vi "asset.update_set_name.vi"(8 "error in":errorcluster, 11 "AssetUpdateStaging in":refnum<class "AssetUpdateStaging.lvclass">) -> (0 "error out":errorcluster, 3 "AssetUpdateStaging out":refnum<class "AssetUpdateStaging.lvclass">)   [LabVIEW 2020, in "AssetUpdateStaging.lvclass"]
doc: "Stages a new name for the asset being updated."
uses:
  AssetUpdateStaging.lvclass
  AssetUpdateStaging.lvclass/AssetUpdateStaging.ctl
  client.lvlib
panel:
  in  "name":string
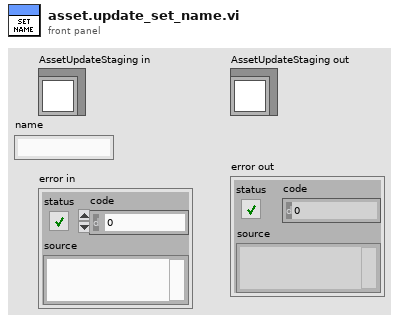
[diagram p1: front panel]
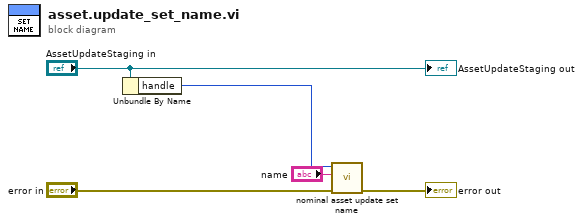
[diagram p0: block diagram]
diagram:
  n1 = Unbundle By Name("AssetUpdateStaging in") -> ("handle"=w3:i32)
  n2 = call "nominal asset update set name.vi"("error in (no error)"="error in", "name"="name", "staging"=w3) -> ("error out"=→"error out":errorcluster)  [unwired: 7 in, 1 out]
  "AssetUpdateStaging out" <- "AssetUpdateStaging in"
